vi "GetMonitorData.vi"(7 "LabVIEW Web Service Request":refnum<class "Web Request.lvclass">, 11 "Channel":i32) -> (3 "LVArray":dbl[][](array[numeric]))   [LabVIEW 2018]
uses:
  <vilib>/wsapi/Web Request.lvclass
  CAEN globals.vi
  <userlib>/_OpenG.lib/array/array.llb/Search 1D Array (I32)__ogtk.vi
  <vilib>/Analysis/Matrix/Numeric/Conversions/Matrix To Array - RM.vi
  <vilib>/Analysis/Matrix/NI_Matrix.lvlib
panel:
  out "error out":errorcluster
  in  "error in (no error)":errorcluster
  # "Use the Web Service Request input terminal to call the VIs on the Web Services palette. Do not remove it from the connector pane unless you don't need access to the palette."
  # "Each additional control wired to the connector pane will be available as an input in the URL. To include an indicator in terminal-mode output (the default setting), it must also be wired to the connector pane."
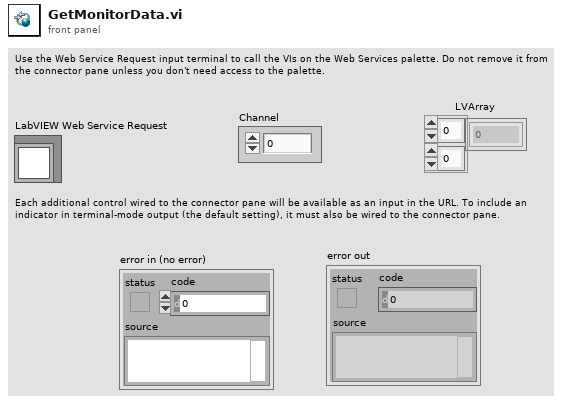
[diagram p1: front panel]
types:
  T1 = typedef "NI_Matrix.lvlib/RealMatrix.ctl" = dbl[][]
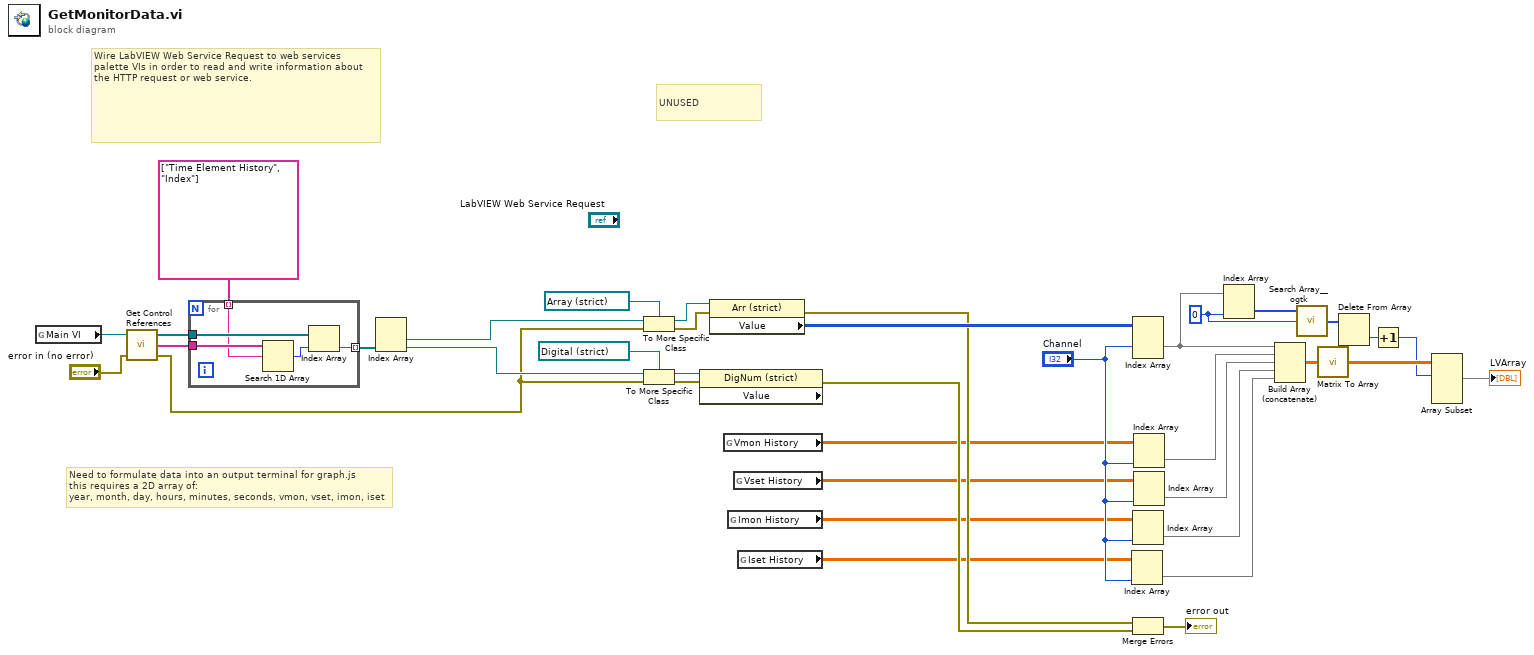
[diagram p0: block diagram]
diagram:
  w6 = 0 ("disabled index (col)")
  # "UNUSED"
  # "Need to formulate data into an output terminal for graph.js\nthis requires a 2D array of:\nyear, month, day, hours, minutes, seconds, vmon, vset, imon, iset"
  # "Wire LabVIEW Web Service Request to web services palette VIs in order to read and write information about the HTTP request or web service."
  n1 = global read "CAEN globals.vi" "Main VI"() -> (w37:refnum<vi>)
  n2 = call "Get Control References.vi"("error in"="error in (no error)", "This vi"=w37) -> ("error out"=w22:errorcluster, "Control Names"=w36:string[], "Controls[]"=w35:refnum<vi>[])  [unwired: 1 in]
  n3 = for {
    tunnel: w36 -> [w42]
    tunnel: w35 -> [w40]
    tunnel: [w39] -> w32 mode=indexing
    tunnel: string[] ["Time Element History", "Index"] ("Control Names") -> [w38] mode=indexing
    n4 = Search 1D Array(1D array=w42, element=w38) -> (index of element=w41:i32)  [unwired: 1 in]
    n5 = Index Array(array=w40, index=w41) -> (element=w39:refnum<vi>)
  }
  n6 = Index Array(array=w32) -> (element #1=w31:refnum<vi>, element #2=w26:refnum<vi>)  [unwired: 2 in]
  n7 = To More Specific Class(target class=refnum<vi> refnum ("Time Element History"), reference=w31, error in=w22) -> (specific class reference=w29:refnum<vi>, error out=w28:errorcluster)
  n8 = To More Specific Class(target class=refnum<vi> refnum ("Channel"), reference=w26, error in=w22) -> (specific class reference=w24:refnum<vi>, error out=w23:errorcluster)
  n9 = property class="DigNum (strict)" props=["Value"](reference=w24, error in=w23) -> (error out=w20:errorcluster)  [unwired: 2 out]
  n10 = property class="Arr (strict)"(reference=w29, error in=w28) -> (error out=w21:errorcluster, "Value"=w27:i32[][][])  [unwired: 1 out]
  n11 = global read "CAEN globals.vi" "Vmon History"() -> (w1:dbl[][])
  n12 = global read "CAEN globals.vi" "Imon History"() -> (w3:dbl[][])
  n13 = global read "CAEN globals.vi" "Vset History"() -> (w2:dbl[][])
  n14 = global read "CAEN globals.vi" "Iset History"() -> (w4:dbl[][])
  n15 = Index Array(array=w4, index (col)="Channel") -> (element=w14:dbl[])  [unwired: 1 in]
  n16 = Index Array(array=w27, index (dim 1)="Channel") -> (element=w12:i32[][])  [unwired: 2 in]
  n17 = Index Array(array=w3, index (col)="Channel") -> (element=w15:dbl[])  [unwired: 1 in]
  n18 = Merge Errors(w21, w20) -> (→"error out":errorcluster)
  n19 = Index Array(array=w1, index (col)="Channel") -> (element=w17:dbl[])  [unwired: 1 in]
  n20 = Index Array(array=w2, index (col)="Channel") -> (element=w16:dbl[])  [unwired: 1 in]
  n21 = Index Array(array=w12, index (col)=w6) -> (element=w7:i32[])  [unwired: 1 in]
  n22 = Build Array (concatenate)(w12, w17, w16, w15, w14) -> (w19:T1)
  n23 = call-poly <userlib>:"Search Array__ogtk.vi"("Array"=w7, "Element Data"=w6) -> ("Indices of Elements"=w9:i32[])  [unwired: 7 in]
  n24 = call-poly <vilib>:"Matrix To Array.vi"("Real Matrix"=w19) -> ("Real 2D Array"=w11:dbl[][])
  n25 = Delete From Array(array=w9) -> (deleted portion=w8:i32)  [unwired: 2 in, 1 out]
  n26 = Increment(x=w8) -> (x+1=w5:i32)
  n27 = Array Subset(array=w11, index (row)=w5) -> (→"LVArray":dbl[][])  [unwired: 3 in]
